vi "Factory.vi"(0 "TTLController in":refnum<class "TTLController.lvclass">, 7 "Variant":variant, 9 "Prefix":string, 11 "error in (no error)":errorcluster) -> (4 "TTLController out":refnum<class "TTLController.lvclass">, 8 "Type":string, 15 "error out":errorcluster)   [LabVIEW 2020, in "TTLController.lvclass"]
uses:
  TTLController.lvclass
  TTLController.lvclass/TTLController.ctl
  TTLWaterController/TTLWaterController.lvclass
  D:/Development/epl-tosca/LV Source/TTL VIs/Control Classes/Base Class/TTLController.lvclass
  TCPController/TCPController.lvclass
  epl-vi-lib/Koop/KObject Class/KObject.lvclass
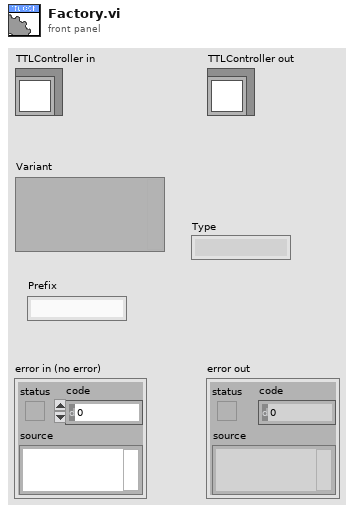
[diagram p1: front panel]
types:
  T1 = typedef "TTLController.lvclass/Serialized.ctl" = cluster{"Name":string, "Start":T2, "Stop":T2, "Pulse":cluster{"Active":bool, "IPI":string, "Width (ms)":dbl}}
  T2 = typedef "TTLController.lvclass/Trigger.ctl" = cluster{"When":string, "Expr":string}
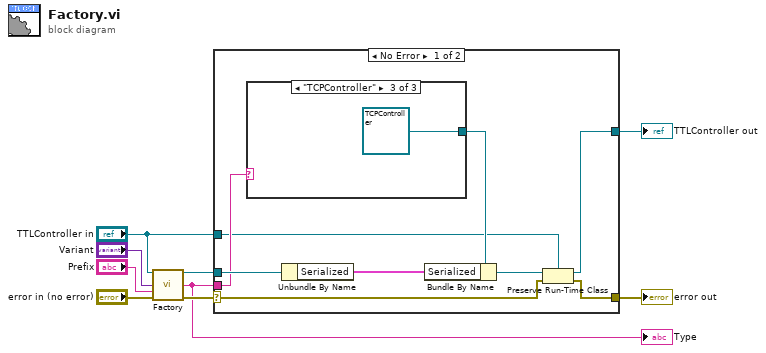
[diagram p0: block diagram]
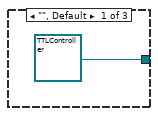
[diagram p2: hidden frame]
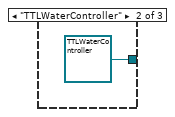
[diagram p3: hidden frame]
diagram:
  n1 = call-parent "Factory.vi"("KObject in"="TTLController in", "Variant"="Variant", "Prefix"="Prefix", "error in (no error)"="error in (no error)") -> ("KObject out"=w4:refnum<class "TTLController.lvclass">, "Type"=w3:string, "error out"=w6:errorcluster)  [unwired: 9 in]
  "Type" <- w3
  n2 = case shown="No Error" w6 {
    selector: w6 -> [w13 w23]
    tunnel: [w12 w23] -> w5
    tunnel: [w10 w22] -> w2
    tunnel: w4 -> [w16 _]
    tunnel: w3 -> [w15 _]
    tunnel: "TTLController in" -> [w11 w22]
    frame No Error {
      n3 = case shown="\"TCPController\"" w15 {
        tunnel: [refnum<class "TTLController.lvclass"> refnum ("TTLControl") refnum<class "TTLWaterController.lvclass"> refnum ("TTLWater") refnum<class "TCPController.lvclass"> refnum ("TCPController")] -> w18
        frame "", Default {
        }
        frame "TTLWaterController" {
        }
        frame "TCPController" {
        }
      }
      n4 = Unbundle By Name(w16) -> ("Serialized"=w17:T1)
      n5 = Bundle By Name(cluster=w18, "Serialized"=w17) -> (w14:refnum<class "TTLController.lvclass">)
      n6 = Preserve Run-Time Class(object in=w14, error in=w13, 2:w11) -> (object out=w10:refnum<class "TTLController.lvclass">, error out=w12:errorcluster)
    }
    frame Error {
    }
  }
  "error out" <- w5
  "TTLController out" <- w2
